vi "RoboRIO-Teensy-ADIS16448-Interface Example.vi"   [LabVIEW 2015]
uses:
  ADIS16448_RoboRIO_Teensy_Interface_Lib/RoboRIO-Teensy-ADIS16448-Interface.lvlib
types:
  T1 = typedef "WPI_SerialPortRef.ctl" = cluster{"DevStatus":errorcluster, "Serial Port Name":refnum<visa-resource-name>}
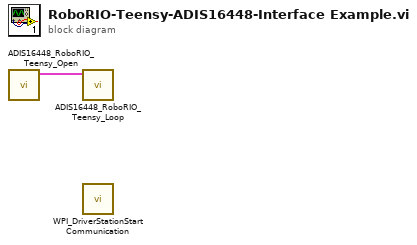
[diagram p0: block diagram]
diagram:
  n1 = call "ADIS16448_RoboRIO_Teensy_Open.vi"() -> ("SerialPortRef"=w1:T1)  [unwired: 9 in, 1 out]
  n2 = call "ADIS16448_RoboRIO_Teensy_Loop.vi"("SerialPortRef"=w1) -> ()  [unwired: 11 in]
  n3 = call <vilib>:"WPI_DriverStationStart Communication.vi"() -> ()  [unwired: 12 in]
